vi "dataUserIn.vi"(8 "error in (no error)":errorcluster, 10 "password":string, 11 "username":string) -> (0 "error out":errorcluster)   [LabVIEW 2014]
panel:
  out "连接的字符串":string
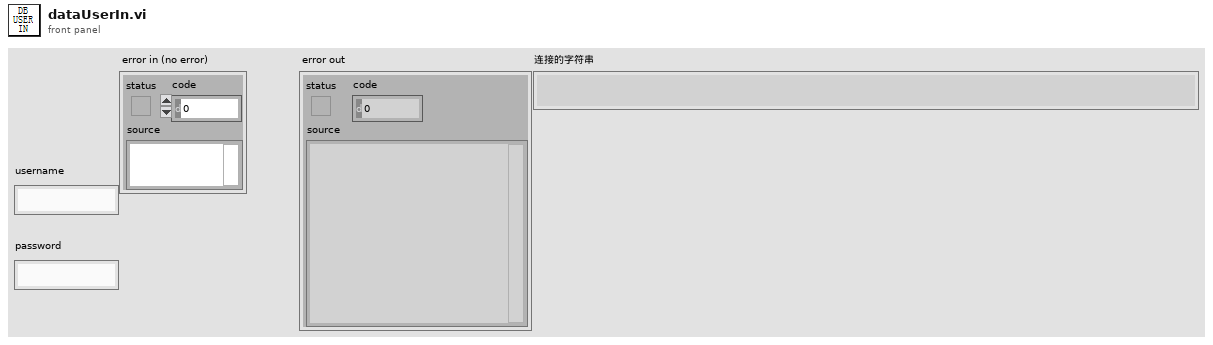
[diagram p1: front panel]
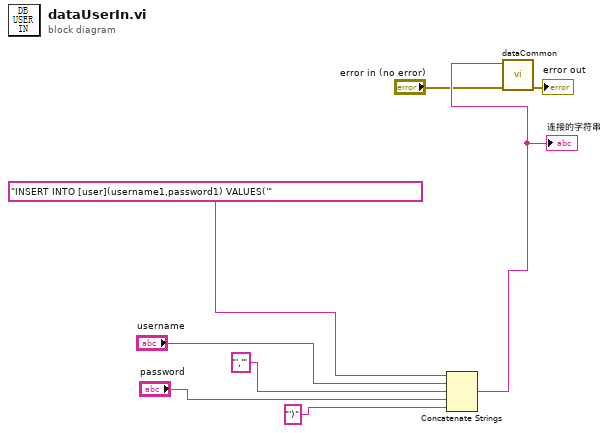
[diagram p0: block diagram]
diagram:
  n1 = Concatenate Strings("INSERT INTO [user](username1,password1) VALUES('", "username", "','", "password", "')") -> (w4:string)
  "连接的字符串" <- w4
  n2 = call "dataCommon.vi"("error in (no error)"="error in (no error)", "Command Text"=w4) -> ("error out"=→"error out":errorcluster)  [unwired: 8 in, 1 out]
